vi "3.模拟IO节点使用.vi"() -> ()   [LabVIEW 2019]
uses:
  <vilib>/rvi/Emulation/niFpgaGetClockAttributes.vi
  <vilib>/rvi/Emulation/niFpgaSctlEmulationGetInTimedLoop.vi
  <vilib>/rvi/Emulation/niFpgaEmulationReportErrorSimple.vi
  <vilib>/rvi/eio/common/nirviEmuTemplateMethod_errors.vi
  <vilib>/rvi/Emulation/niFpgaCriticalErrorInLSC.vi
  <vilib>/eio/EIONode/EIONode.xnode
panel:
  out "布尔":bool
  in  "阈值":fxp<+/-,24,5>=3.0
  out "ConnectorA/AI0":fxp<+/-,24,5>
  in  "ConnectorA/AO0":sgl(slide) scale=1.0..5.0
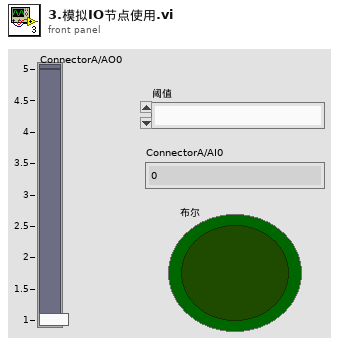
[diagram p1: front panel]
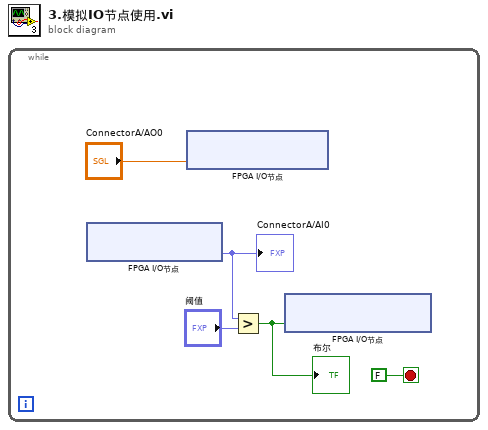
[diagram p0: block diagram]
diagram:
  n1 = while {
    stop <- FALSE stop-if-true
    n2 = xnode "FPGA I/O节点"() -> ("ConnectorA/AI0"=w3:fxp<+/-,24,5>)  [unwired: 1 in, 1 out]
    "ConnectorA/AI0" <- w3
    n3 = xnode "FPGA I/O节点"("ConnectorA/AO0"="ConnectorA/AO0") -> ()  [unwired: 1 in, 1 out]
    n4 = Greater?(x=w3, y="阈值") -> (0:w1:bool)
    "布尔" <- w1
    n5 = xnode "FPGA I/O节点"("ConnectorA/DIO0"=w1) -> ()  [unwired: 1 in, 1 out]
  }
